vi "Read.vi"(8 "error in (no error)":errorcluster, 9 "Starting independent variables":dbl[](array[numeric]), 10 "Current independent variables":dbl[](array[numeric]), 11 "PC Reader in":refnum<class "PC Reader.lvclass">) -> (0 "error out":errorcluster, 2 "Data Channels":T1, 3 "PC Reader out":refnum<class "PC Reader.lvclass">)   [LabVIEW 2017, in "PC Reader.lvclass"]
doc: "Prepare for read, wait the time delay, and take data from up to 4 channels."
uses:
  PC Reader.lvclass
  Instruments/Photon Counter/SR400/SR400.lvlib
  Instruments/Utility Classes/Readable/X.ctl
  Instruments/Utility Classes/Readable/Readable.lvclass
  Reader/Reader.lvclass
  Instruments/Utility Classes/Readable/Data Point.ctl
  Instruments/Utility Classes/Readable/Data Channel.ctl
  Instruments/Utility Classes/Readable/Data Channels.ctl
  Instruments/Utility Classes/Readable/Time.ctl
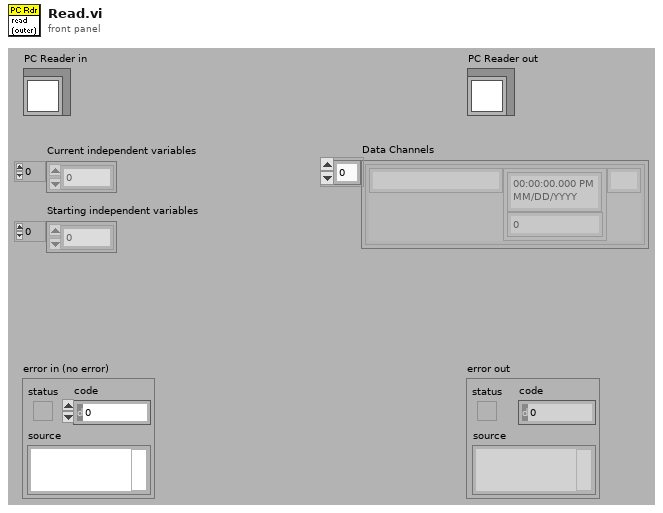
[diagram p1: front panel]
types:
  T1 = typedef "Readable.lvclass/Data Channels.ctl" = T2[]
  T2 = typedef "Readable.lvclass/Data Channel.ctl" = cluster{"Name":string, "Data Point":T3, "Unit":string}
  T3 = typedef "Readable.lvclass/Data Point.ctl" = cluster{"t":T4, "x":T5}
  T4 = typedef "Readable.lvclass/Time.ctl" = timestamp
  T5 = typedef "Readable.lvclass/X.ctl" = dbl
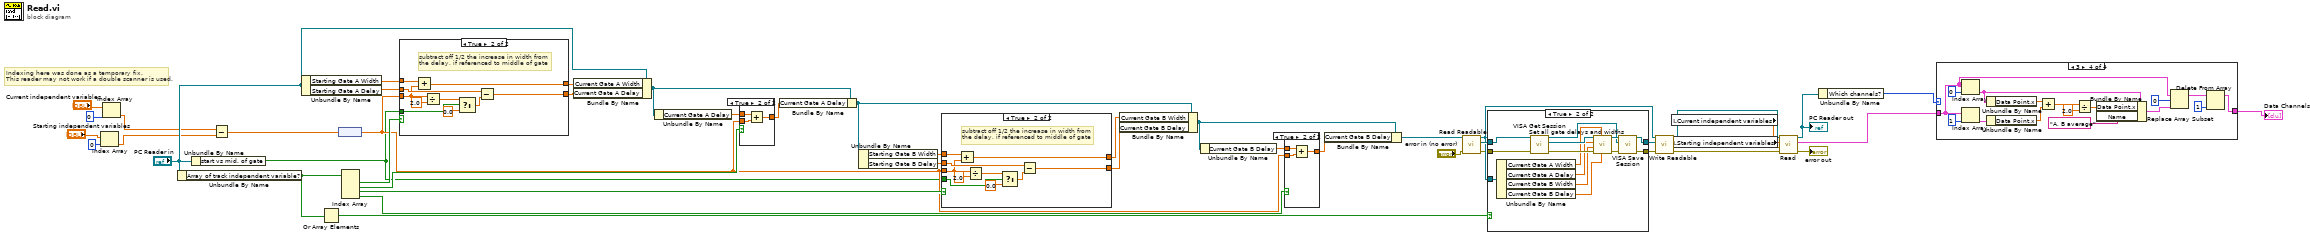
[diagram p0: block diagram]
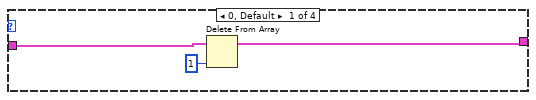
[diagram p2: hidden frame]
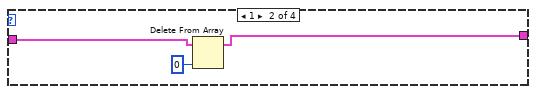
[diagram p3: hidden frame]
diagram:
  # "Indexing here was done as a temporary fix.\nThis reader may not work if a double scanner is used."
  n1 = Index Array(array="Starting independent variables", index=0) -> (element=w2:dbl)
  n2 = Index Array(array="Current independent variables", index=0) -> (element=w1:dbl)
  n3 = Unbundle By Name("PC Reader in") -> ("Array of track independent variable?"=w18:bool[])
  n4 = Unbundle By Name("PC Reader in") -> ("start vs mid. of gate"=w23:bool)
  n5 = Subtract(x=w1, y=w2) -> (x-y=w19:dbl)
  n6 = Unbundle By Name("PC Reader in") -> ("Starting Gate A Width"=w44:dbl[unit], "Starting Gate A Delay"=w27:dbl[unit])
  n7 = Or Array Elements(Boolean array=w18) -> (logical OR=w17:bool)
  n8 = node(w19) -> (w35:dbl[unit])
  n9 = Index Array(array=w18) -> (element #1=w36:bool, element #2=w47:bool, element #3=w46:bool, element #4=w45:bool)  [unwired: 4 in]
  n10 = case shown="True" w36 {
    tunnel: w35 -> [_ w50]
    tunnel: w44 -> [w49 w59]
    tunnel: [w49 w53] -> w28
    tunnel: w23 -> [_ w57]
    tunnel: w27 -> [w48 w55]
    tunnel: [w48 w51] -> w26
    frame False {
    }
    frame True {
      # "subtract off 1/2 the increase in width from \nthe delay, if referenced to middle of gate"
      n11 = Add(x=w59, y=w50) -> (x+y=w53:dbl[unit])
      n12 = Divide(x=w50, y=2.0) -> (x/y=w52:dbl[unit])
      n13 = Select(t=w52, s=w57, f=dbl[unit] 0.0) -> (s? t:f=w58:dbl[unit])
      n14 = Subtract(x=w55, y=w58) -> (x-y=w51:dbl[unit])
    }
  }
  n15 = Bundle By Name(cluster="PC Reader in", "Current Gate A Width"=w28, "Current Gate A Delay"=w26) -> (w31:refnum<class "PC Reader.lvclass">)
  n16 = Unbundle By Name(w31) -> ("Current Gate A Delay"=w37:dbl[unit])
  n17 = case shown="True" w47 {
    tunnel: w35 -> [_ w62]
    tunnel: w37 -> [w60 w61]
    tunnel: [w60 w63] -> w34
    frame False {
    }
    frame True {
      n18 = Add(x=w61, y=w62) -> (x+y=w63:dbl[unit])
    }
  }
  n19 = Bundle By Name(cluster=w31, "Current Gate A Delay"=w34) -> (w30:refnum<class "PC Reader.lvclass">)
  n20 = Unbundle By Name(w30) -> ("Starting Gate B Width"=w38:dbl[unit], "Starting Gate B Delay"=w24:dbl[unit])
  n21 = case shown="True" w46 {
    tunnel: w35 -> [_ w66]
    tunnel: w38 -> [w65 w75]
    tunnel: [w65 w68] -> w33
    tunnel: [w64 w71] -> w25
    tunnel: w24 -> [w64 w70]
    tunnel: w23 -> [_ w69]
    frame False {
    }
    frame True {
      # "subtract off 1/2 the increase in width from \nthe delay, if referenced to middle of gate"
      n22 = Add(x=w75, y=w66) -> (x+y=w68:dbl[unit])
      n23 = Divide(x=w66, y=2.0) -> (x/y=w67:dbl[unit])
      n24 = Select(t=w67, s=w69, f=dbl[unit] 0.0) -> (s? t:f=w72:dbl[unit])
      n25 = Subtract(x=w70, y=w72) -> (x-y=w71:dbl[unit])
    }
  }
  n26 = Bundle By Name(cluster=w30, "Current Gate B Width"=w33, "Current Gate B Delay"=w25) -> (w29:refnum<class "PC Reader.lvclass">)
  n27 = Unbundle By Name(w29) -> ("Current Gate B Delay"=w39:dbl[unit])
  n28 = case shown="True" w45 {
    tunnel: w35 -> [_ w77]
    tunnel: w39 -> [w76 w78]
    tunnel: [w76 w79] -> w32
    frame False {
    }
    frame True {
      n29 = Add(x=w78, y=w77) -> (x+y=w79:dbl[unit])
    }
  }
  n30 = Bundle By Name(cluster=w29, "Current Gate B Delay"=w32) -> (w14:refnum<class "PC Reader.lvclass">)
  n31 = call-dynamic "Read Readable.vi"("error in (no error)"="error in (no error)", "Reader.lvclass in"=w14) -> ("error out"=w12:errorcluster, "Readable.lvclass"=w22:refnum<class "Readable.lvclass">, "Reader.lvclass out"=w15:refnum<class "PC Reader.lvclass">)  [unwired: 7 out]
  n32 = case shown="True" w17 {
    tunnel: w22 -> [w81 w95]
    tunnel: [w81 w94] -> w21
    tunnel: w12 -> [w80 w92]
    tunnel: [w80 w91] -> w20
    tunnel: w15 -> [_ w90]
    frame False {
    }
    frame True {
      n33 = Unbundle By Name(w90) -> ("Current Gate A Width"=w85:dbl[unit], "Current Gate A Delay"=w84:dbl[unit], "Current Gate B Width"=w83:dbl[unit], "Current Gate B Delay"=w82:dbl[unit])
      n34 = call-dynamic "VISA Get Session.vi"("error in (no error)"=w92, "Instrument.lvclass in"=w95) -> ("error out"=w87:errorcluster, "VISA Resource Name"=w89:refnum<visa-resource-name>, "Instrument.lvclass out"=w93:refnum<class "Readable.lvclass">)  [unwired: 7 out]
      n35 = call "Set all gate delays and widths.vi"("Gate B Delay (def: 0 s)"=w82, "Gate A Width (def: 0 s)"=w85, "error in (no error)"=w87, "Gate B Width (def: 0 s)"=w83, "Gate A Delay (def: 0 s)"=w84, "VISA resource name"=w89) -> ("error out"=w86:errorcluster, "VISA resource name out"=w88:refnum<visa-resource-name>)  [unwired: 4 out]
      n36 = call-dynamic "VISA Save Session.vi"("error in (no error)"=w86, "VISA Resource Name"=w88, "Instrument.lvclass in"=w93) -> ("error out"=w91:errorcluster, "Instrument.lvclass out"=w94:refnum<class "Readable.lvclass">)  [unwired: 7 out]
    }
  }
  n37 = call-dynamic "Write Readable.vi"("error in (no error)"=w20, "Readable.lvclass"=w21, "Reader.lvclass in"=w15) -> ("error out"=w43:errorcluster, "Reader.lvclass out"=w42:refnum<class "PC Reader.lvclass">)  [unwired: 7 out]
  n38 = local read "Current independent variables"() -> (w41:dbl[])
  n39 = local read "Starting independent variables"() -> (w40:dbl[])
  n40 = call-parent "Read.vi"("error in (no error)"=w43, "Starting independent variables"=w40, "Current independent variables"=w41, "Reader in"=w42) -> ("error out"=→"error out":errorcluster, "Data Channels"=w8:T1, "Reader out"=w9:refnum<class "PC Reader.lvclass">)  [unwired: 5 out]
  "PC Reader out" <- w9
  n41 = Unbundle By Name(w9) -> ("Which channels?"=w10:u16)
  n42 = case shown="3" w10 {
    tunnel: w8 -> [w98 w101 w102 w105]
    tunnel: [w96 w99 w102 w106] -> w7
    frame 0, Default {
      n43 = Delete From Array(array=w98, index=1) -> (array with subset deleted=w96:T1)  [unwired: 1 in, 1 out]
    }
    frame 1 {
      n44 = Delete From Array(array=w101, index=0) -> (array with subset deleted=w99:T1)  [unwired: 1 in, 1 out]
    }
    frame 2 {
    }
    frame 3 {
      n45 = Index Array(array=w105, index=0) -> (element=w111:T2)
      n46 = Index Array(array=w105, index=1) -> (element=w116:T2)
      n47 = Unbundle By Name(w111) -> ("Data Point.x"=w115:T5)
      n48 = Unbundle By Name(w116) -> ("Data Point.x"=w114:T5)
      n49 = Add(x=w115, y=w114) -> (x+y=w113:T5)
      n50 = Divide(x=w113, y=T5 2.0) -> (x/y=w110:T5)
      n51 = Bundle By Name(cluster=w111, "Data Point.x"=w110, "Name"="A, B average") -> (w108:T2)
      n52 = Replace Array Subset(array=w105, new element=w108, index=0) -> (w107:T1)
      n53 = Delete From Array(array=w107, index=1) -> (array with subset deleted=w106:T1)  [unwired: 1 in, 1 out]
    }
  }
  "Data Channels" <- w7
